vi "UIManager.CreateBroadcasts.vi"(8 "error in (no error)":errorcluster) -> (0 "error out":errorcluster, 3 "Broadcasts":T1)   [LabVIEW 2024, in "UIManager.lvclass"]
uses:
  UIManager.lvclass
  UIManager.lvclass/UIManager.ctl
  Stopped.ctl
  Broadcast Events--cluster.ctl
  RQMHCore/ModuleCore/Module.lvclass
  Request Stop.ctl
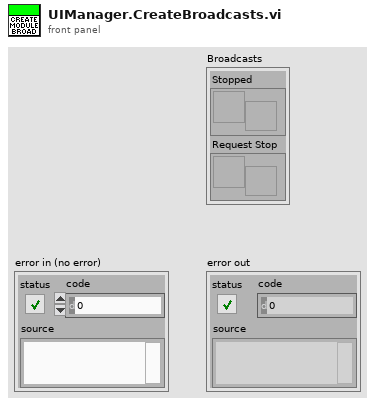
[diagram p1: front panel]
types:
  T1 = typedef "UIManager.lvclass/Broadcast Events--cluster.ctl" = cluster{"Stopped":refnum<user-event>, "Request Stop":refnum<user-event>}
  T2 = typedef "UIManager.lvclass/Request Stop.ctl" = cluster{"Module":refnum<class "Module.lvclass">, "Critical":bool}
  T3 = typedef "UIManager.lvclass/Stopped.ctl" = bool
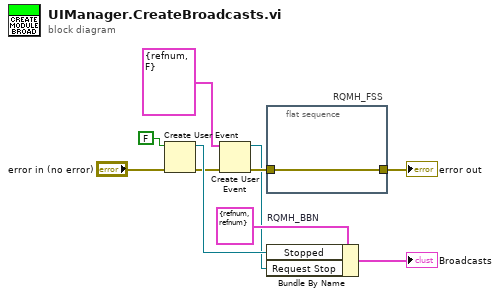
[diagram p0: block diagram]
diagram:
  n1 = Create User Event(user event datatype=T3 FALSE ("Stopped"), error in="error in (no error)") -> (user event=w9:refnum<user-event>, error out=w4:errorcluster)
  n2 = Create User Event(user event datatype=T2 {"Module"=refnum, "Critical"=FALSE} ("Request Stop"), error in=w4) -> (user event=w1:refnum<user-event>, error out=w3:errorcluster)
  n3 = flat-sequence "RQMH_FSS" {
    tunnel: w3 -> [w11]
    tunnel: [w11] -> w5
    frame #0 {
    }
  }
  n4 = Bundle By Name "RQMH_BBN"(cluster=T1 {"Stopped"=refnum, "Request Stop"=refnum} ("Broadcasts"), "Stopped"=w9, "Request Stop"=w1) -> (→"Broadcasts":T1)
  "error out" <- w5
